vi "MXG_Set_ARB_Sample_Rate.vi"(0 "VISA resource name":refnum<visa-resource-name>, 9 "ARB Sample Rate":dbl, 11 "error in":errorcluster) -> (4 "VISA resource name":refnum<visa-resource-name>, 15 "error out":errorcluster)   [LabVIEW 2016]
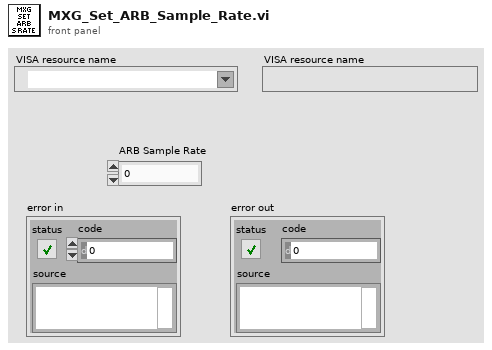
[diagram p1: front panel]
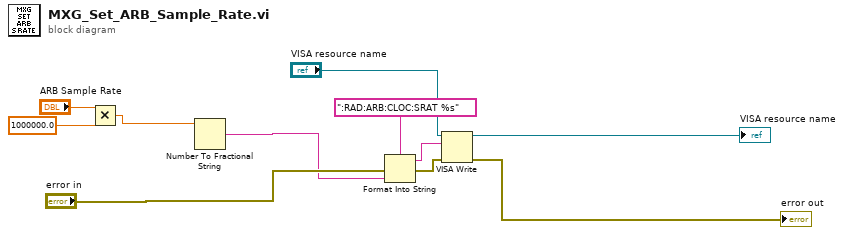
[diagram p0: block diagram]
diagram:
  n1 = Multiply(x="ARB Sample Rate", y=1000000.0) -> (x*y=w1:dbl)
  n2 = Number To Fractional String(number=w1) -> (F-format string=w4:string)  [unwired: 3 in]
  n3 = Format Into String(format string=":RAD:ARB:CLOC:SRAT %s", error in="error in", w4) -> (resulting string=w8:string, error out=w10:errorcluster)  [unwired: 1 in]
  n4 = VISA Write(VISA resource name="VISA resource name", write buffer=w8, error in (no error)=w10) -> (VISA resource name out=→"VISA resource name":refnum<visa-resource-name>, error out=→"error out":errorcluster)  [unwired: 1 out]
